vi "nominal ingest parquet new dataset.vi"(6 "out_job":i32, 7 "dataset_create":i32, 8 "error in (no error)":errorcluster, 9 "file_path":string, 10 "staging":i32, 11 "client":i32) -> (0 "error out":errorcluster, 3 "function return":i32, 4 "out_job out":i32)   [LabVIEW 2020, in "client.lvlib"]
doc: "int32_t nominal_ingest_parquet_new_dataset(int32_t client,\n int32_t staging,\n const char *file_path,\n int32_t dataset_create,\n int32_t *out_job);"
uses:
  client.lvlib
  bin/nominalClient_64.dll
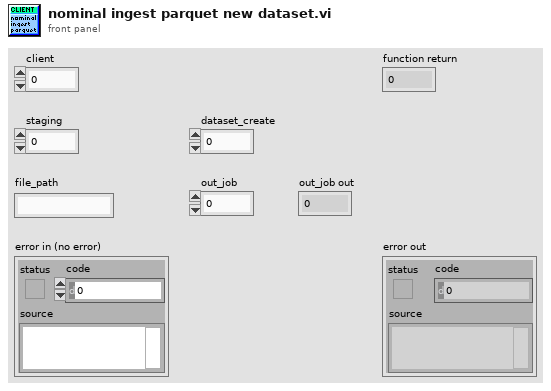
[diagram p1: front panel]
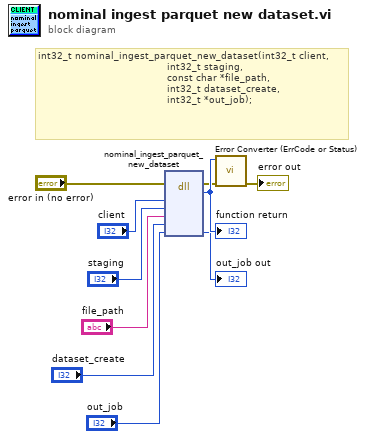
[diagram p0: block diagram]
diagram:
  # "int32_t nominal_ingest_parquet_new_dataset(int32_t client,\n                                           int32_t staging,\n                                           const char *file_path,\n                                           int32_t dataset_create,\n                                           int32_t *out_job);"
  n1 = dll-call lib="C:/code/labview-client-rs/lv_src/bin/nominalClient_*.*" fn="nominal_ingest_parquet_new_dataset"(error in="error in (no error)", "client"="client", "staging"="staging", "file_path"="file_path", "dataset_create"="dataset_create", "out_job"="out_job") -> (error out=w2:errorcluster, w10:i32, "out_job"=→"out_job out":i32)  [unwired: 6 in, 1 out]
  "function return" <- w10
  n2 = call "Error Converter (ErrCode or Status).vi"("error in (no error)"=w2, "error code"=w10) -> ("error out"=→"error out":errorcluster)  [unwired: 9 in]
